vi "Evaluation_intensity.vi"(1 "X1":sgl, 2 "DataXY":cluster{"X array":dbl[], "Y array":dbl[]}) -> (0 "Y intensity":sgl)   [LabVIEW 2010]
uses:
  <vilib>/gmath/NI_Gmath.lvlib
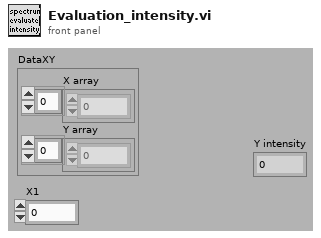
[diagram p1: front panel]
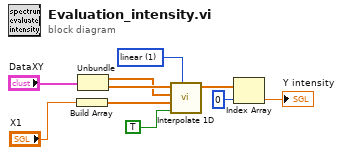
[diagram p0: block diagram]
diagram:
  w1 = 1 items=["nearest", "linear", "spline", "cubic Hermite", "Lagrange"] ("method")
  n1 = Build Array("X1") -> (w6:sgl[])
  n2 = Unbundle("DataXY") -> ("X array"=w8:dbl[], "Y array"=w9:dbl[])
  n3 = call <vilib>:"Interpolate 1D.vi"("method"=w1, "X is monotonic"=TRUE, "xi"=w6, "X"=w8, "Y"=w9) -> ("yi"=w4:dbl[])  [unwired: 4 in, 2 out]
  n4 = Index Array(array=w4, index=0) -> (element=→"Y intensity":dbl)
